vi "Read Channel.vi"(8 "error in (no error)":errorcluster, 11 "Channel in":refnum<class "Channel.lvclass">) -> (0 "error out":errorcluster, 1 "units":string, 2 "name":string, 3 "Channel out":refnum<class "Channel.lvclass">, 4 "index":i32, 5 "type":T1)   [LabVIEW 2017, in "Scan Engine Scripting.lvlib" / "Channel.lvclass"]
doc: "Reads the name, units, index and type of a channel."
uses:
  Channel.lvclass
  Type.ctl
  Channel.lvclass/Channel.ctl
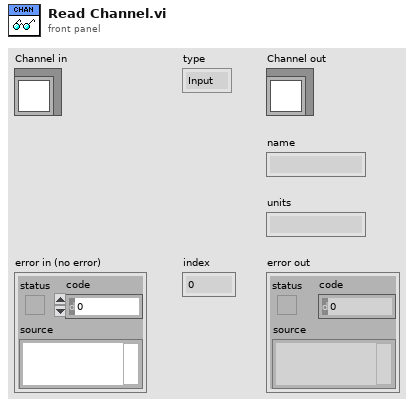
[diagram p1: front panel]
types:
  T1 = typedef "Scan Engine Scripting.lvlib/Channel.lvclass/Type.ctl" = enum16{"Input", "Output"}
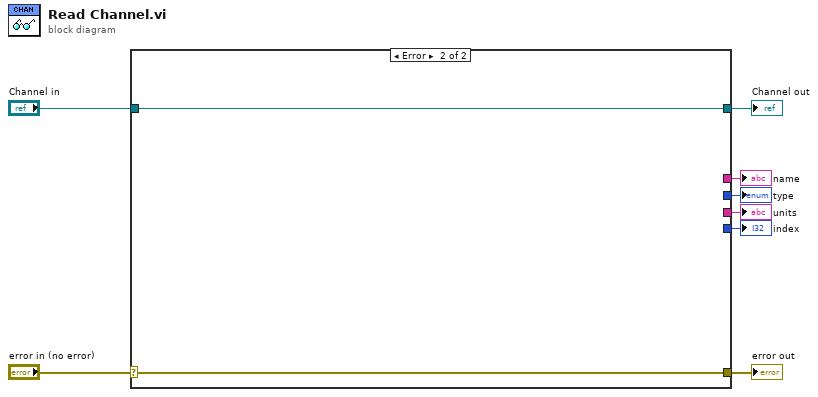
[diagram p0: block diagram]
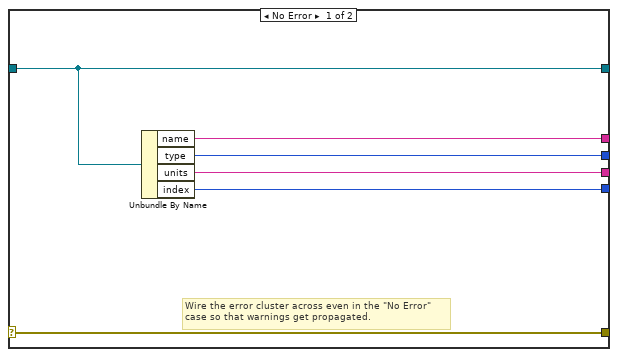
[diagram p2: hidden frame]
diagram:
  n1 = case shown="Error" "error in (no error)" {
    selector: "error in (no error)" -> [w14 w16]
    tunnel: [w14 w16] -> w7
    tunnel: [w13 w15] -> w5
    tunnel: "Channel in" -> [w13 w15]
    tunnel: [w12 _] -> w4
    tunnel: [w11 _] -> w3
    tunnel: [w10 _] -> w2
    tunnel: [w9 _] -> w1
    frame No Error {
      # "Wire the error cluster across even in the \"No Error\"\ncase so that warnings get propagated."
      n2 = Unbundle By Name(w13) -> ("name"=w12:string, "type"=w10:T1, "units"=w9:string, "index"=w11:i32)
    }
    frame Error {
    }
  }
  "error out" <- w7
  "Channel out" <- w5
  "name" <- w4
  "index" <- w3
  "type" <- w2
  "units" <- w1
